vi "Set Current Limit & Limit Range.vi"(8 "error in":errorcluster, 9 "Current Limit Range (A)":dbl format="%#_6p", 10 "Current Limit (A)":dbl format="%#_6p", 11 "DCPower SSC in":T1[](array[typedef])) -> (0 "error out":errorcluster, 3 "DCPower SSC out":T1[](array[typedef]))   [LabVIEW 2019]
uses:
  Instrument Control/DCPower/SSC DCPower/SSC DCPower.ctl
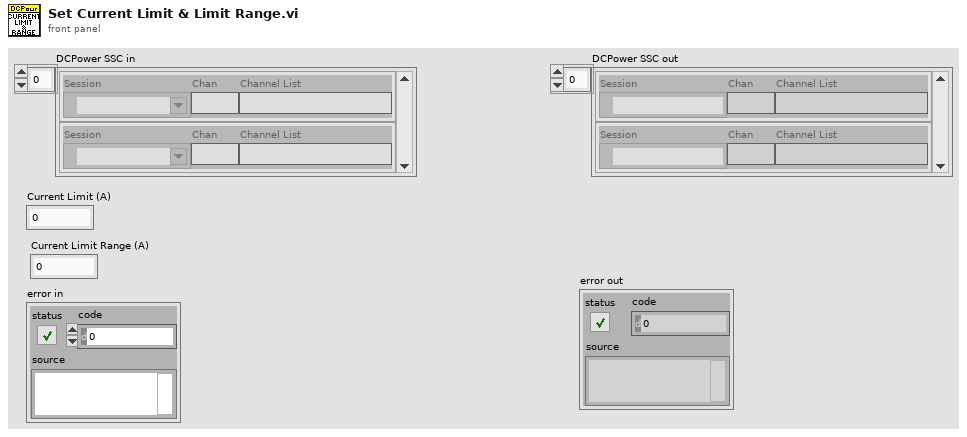
[diagram p1: front panel]
types:
  T1 = typedef "SSC DCPower.ctl" = cluster{"Session":refnum<k15>, "Chan":string, "Channel List":string}
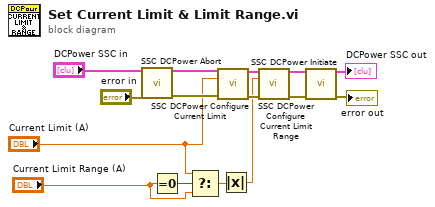
[diagram p0: block diagram]
diagram:
  n1 = call "SSC DCPower Abort.vi"("DCPower SSC in"="DCPower SSC in", "error in"="error in") -> ("DCPower SSC out"=w11:T1[], "error out"=w10:errorcluster)  [unwired: 12 in]
  n2 = Equal To 0?(x="Current Limit Range (A)") -> (x = 0?=w5:bool)
  n3 = Select(t="Current Limit (A)", s=w5, f="Current Limit Range (A)") -> (s? t:f=w4:dbl)
  n4 = call "SSC DCPower Configure Current Limit.vi"("DCPower SSC in"=w11, "Current Limit (A)"="Current Limit (A)", "error in"=w10) -> ("DCPower SSC out"=w14:T1[], "error out"=w12:errorcluster)  [unwired: 11 in]
  n5 = Absolute Value(x=w4) -> (abs(x)=w1:dbl)
  n6 = call "SSC DCPower Configure Current Limit Range.vi"("DCPower SSC in"=w14, "Current Limit Range (A)"=w1, "error in"=w12) -> ("DCPower SSC out"=w15:T1[], "error out"=w13:errorcluster)  [unwired: 11 in]
  n7 = call "SSC DCPower Initiate.vi"("DCPower SSC in"=w15, "error in"=w13) -> ("DCPower SSC out"=→"DCPower SSC out":T1[], "error out"=→"error out":errorcluster)  [unwired: 12 in]
